vi "Get DAQmx Product name.vi"(11 "DAQmx resource name":string) -> (3 "DAQmx product type":string)   [LabVIEW 2021]
uses:
  <resource>/objmgr/daqmx.rc
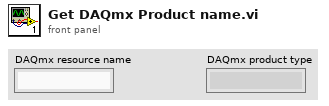
[diagram p1: front panel]
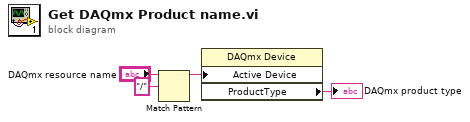
[diagram p0: block diagram]
diagram:
  n1 = Match Pattern(string="DAQmx resource name", regular expression="/") -> (before substring=w3:string)  [unwired: 1 in, 3 out]
  n2 = property class="DAQmx Device"("Active Device"=w3) -> ("ProductType"=→"DAQmx product type":string)  [unwired: 2 in, 2 out]
